vi "Current Display Mouse.vi"(0 "Event Type":T1=enum."Value Change", 2 "Action":T2, 11 "IMAQ Image Display Ref":refnum<vi>) -> (4 "Event Type Out":T1=enum."Value Change", 15 "IMAQ Image Display Ref Out":refnum<vi>)   [LabVIEW 2020]
uses:
  <vilib>/event_ctls.llb/lveventtype.ctl
  Hardware Configuration/Hardware Configuration Controls/Standard Action.ctl
panel:
  out "Channel 5":T3(plugin-control)
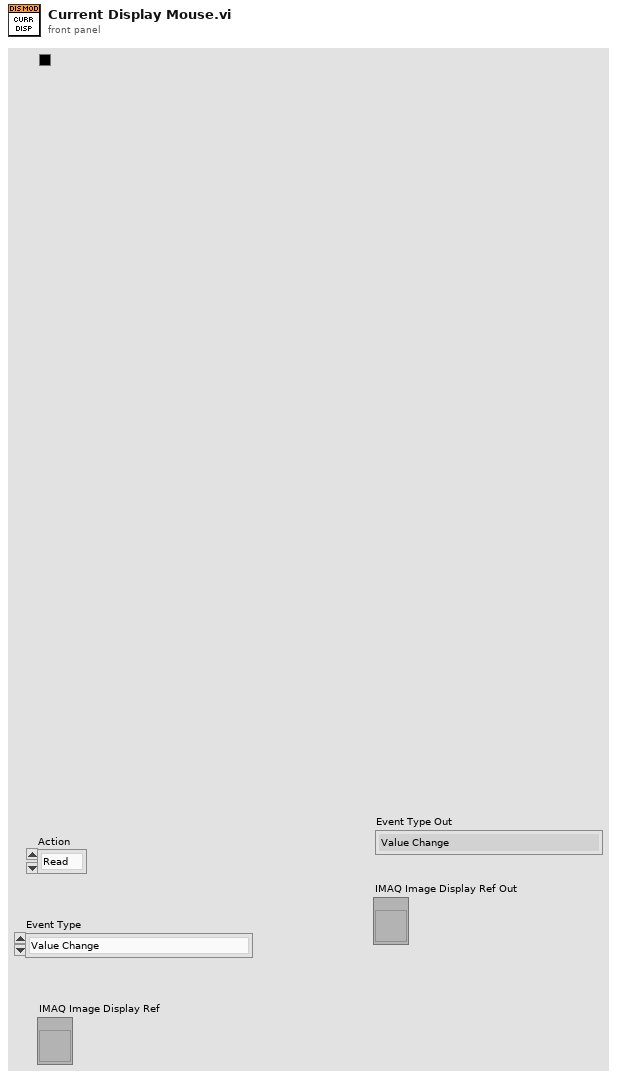
[diagram p1: front panel]
types:
  T1 = typedef "lveventtype.ctl" = enum32{"Null", "Timeout", "Annotation Menu Selection", "Annotation Menu Selection?", "App Instance Close", "App Instance Close?", "Autoscale Range Change", "Bookmark Info Change", "Cell Edit", "Cell Edit?", "Cursor Grab", "Cursor Grab?", "Cursor Menu Selection", "Cursor Menu Selection?", "Cursor Move", "Cursor Release", "Data Change", "Direction Change", "Display State Change", "Drag Ended", "Drag Enter", "Drag Leave", "Drag Over", "Drag Source Update", "Drag Starting", "Drag Starting?", "Drop", "Exec State Change", "Key Down", "Key Down?", "Key Repeat", "Key Repeat?", "Key Up", "Listbox Double Click", "Menu Activation?", "Menu Selection (App)", "Menu Selection? (App)", "Menu Selection (User)", "Mouse Down", "Mouse Down?", "Mouse Enter", "Mouse Leave", "Mouse Move", "Mouse Up", "Mouse Wheel", "NI Security User Change (App)", "Pane Size", "Panel Close", "Panel Close?", "Panel Resize", "Plot Attribute Change", "Scale Range Change", "Shortcut Menu Activation?", "Shortcut Menu Selection (App)", "Shortcut Menu Selection? (App)", "Shortcut Menu Selection (User)", "Tree Double Click", "Tree Drag", "Tree Drag?", "Tree Drop", "Tree Drop?", "Tree Item Close", "Tree Item Close?", "Tree Item Open", "Tree Item Open?", "User Event", "Value Change"}
  T2 = typedef "Standard Action.ctl" = enum16{"Read", "Write"}
  T3 = typedef "IMAQ Image.ctl" = refnum<image>
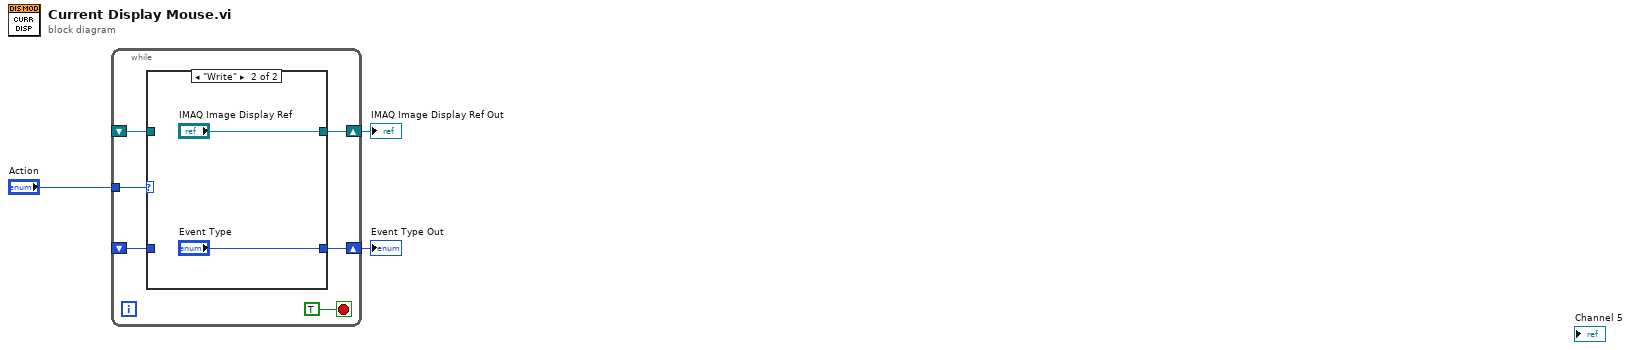
[diagram p0: block diagram]
diagram:
  n1 = while {
    tunnel: "Action" -> [w9]
    shift-right: [w7] -> w2
    shift-left: _ -> [w4]
    shift-right: [w8] -> w1
    shift-left: _ -> [w5]
    stop <- TRUE stop-if-true
    n2 = case shown="\"Write\"" w9 {
      tunnel: [w11 "IMAQ Image Display Ref"] -> w8
      tunnel: [w10 "Event Type"] -> w7
      tunnel: w5 -> [w11 _]
      tunnel: w4 -> [w10 _]
      frame "Read", Default {
      }
      frame "Write" {
      }
    }
  }
  "Event Type Out" <- w2
  "IMAQ Image Display Ref Out" <- w1
